vi "Update Configuration.vi"(8 "error in (no error)":errorcluster, 9 "Config.lvclass":refnum<class "Config.lvclass">, 10 "Config name":T1, 11 "Control in":refnum<class "Control-Server.lvclass">) -> (0 "error out":errorcluster, 3 "Control out":refnum<class "Control-Server.lvclass">)   [LabVIEW 2015, in "Control-Server.lvclass"]
uses:
  Control-Server.lvclass
  Config/config_names_def.ctl
  Config/Config.lvclass
  Control-Server.lvclass/Control-Server.ctl
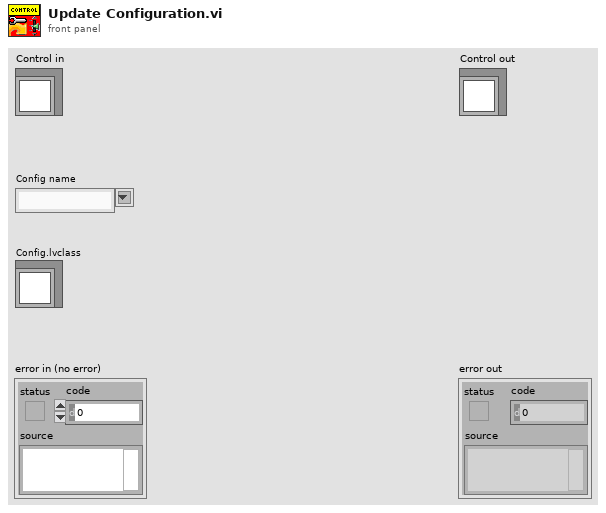
[diagram p1: front panel]
types:
  T1 = typedef "Config.lvclass/config_names_def.ctl" = string
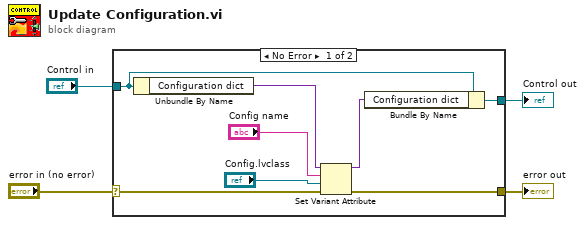
[diagram p0: block diagram]
diagram:
  n1 = case shown="No Error" "error in (no error)" {
    selector: "error in (no error)" -> [w9 w14]
    tunnel: [w8 w14] -> w3
    tunnel: [w6 w13] -> w1
    tunnel: "Control in" -> [w7 w13]
    frame No Error {
      n2 = Unbundle By Name(w7) -> ("Configuration dict"=w12:variant)
      n3 = Set Variant Attribute(Variant=w12, name="Config name", value="Config.lvclass", error in=w9) -> (Variant out=w10:variant, error out=w8:errorcluster)  [unwired: 1 out]
      n4 = Bundle By Name(cluster=w7, "Configuration dict"=w10) -> (w6:refnum<class "Control-Server.lvclass">)
    }
    frame Error {
    }
  }
  "error out" <- w3
  "Control out" <- w1
